vi "Read Compatible Hardware Types.vi"(8 "error in (no error)":errorcluster, 11 "Prototype Measurement in":refnum<class "Prototype Measurement.lvclass">) -> (0 "error out":errorcluster, 2 "Compatible Hardware Types":string[](array[string]), 3 "Prototype Measurement out":refnum<class "Prototype Measurement.lvclass">)   [LabVIEW 2016, in "Prototype Measurement.lvclass"]
uses:
  Prototype Measurement.lvclass
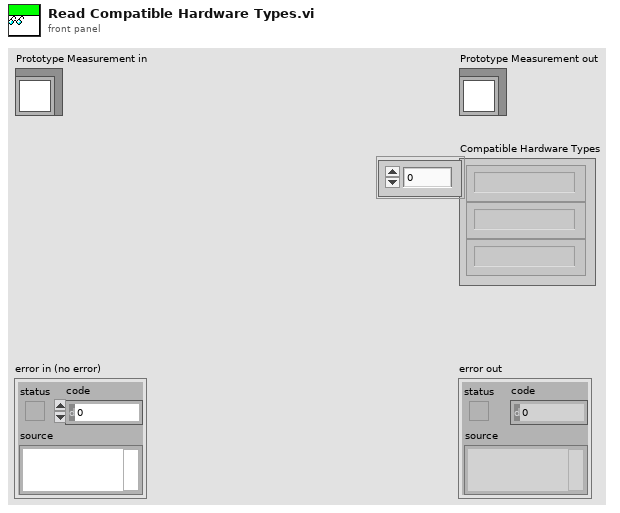
[diagram p1: front panel]
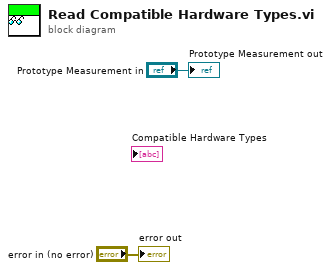
[diagram p0: block diagram]
diagram:
  "error out" <- "error in (no error)"
  "Prototype Measurement out" <- "Prototype Measurement in"
